vi "vacuum tray test.vi"() -> ()   [LabVIEW 2016]
uses:
  Classes/Controllers/I-O/Copy of NI-DAQ Folder/NI-DAQ.lvclass
  D:/INTT/V1/Classes/Controllers/I-O/Copy of I-O Folder/I-O.lvclass
  Classes/Controllers/I-O/Copy of I-O Folder/I-O.lvclass
panel:
  in  "stop":bool
  in  "Values":bool[](array[boolean])=[FALSE, FALSE]
  in  "TrayVaccum":bool
  in  "sampel vacuum":i32[](array[numeric])=[15, 19]
  out "vacuum on?":bool[](array[boolean])
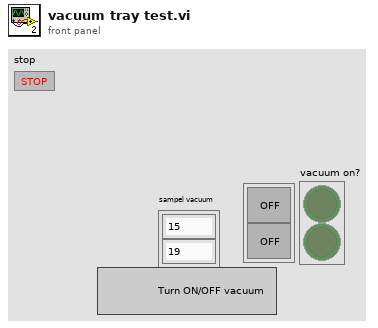
[diagram p1: front panel]
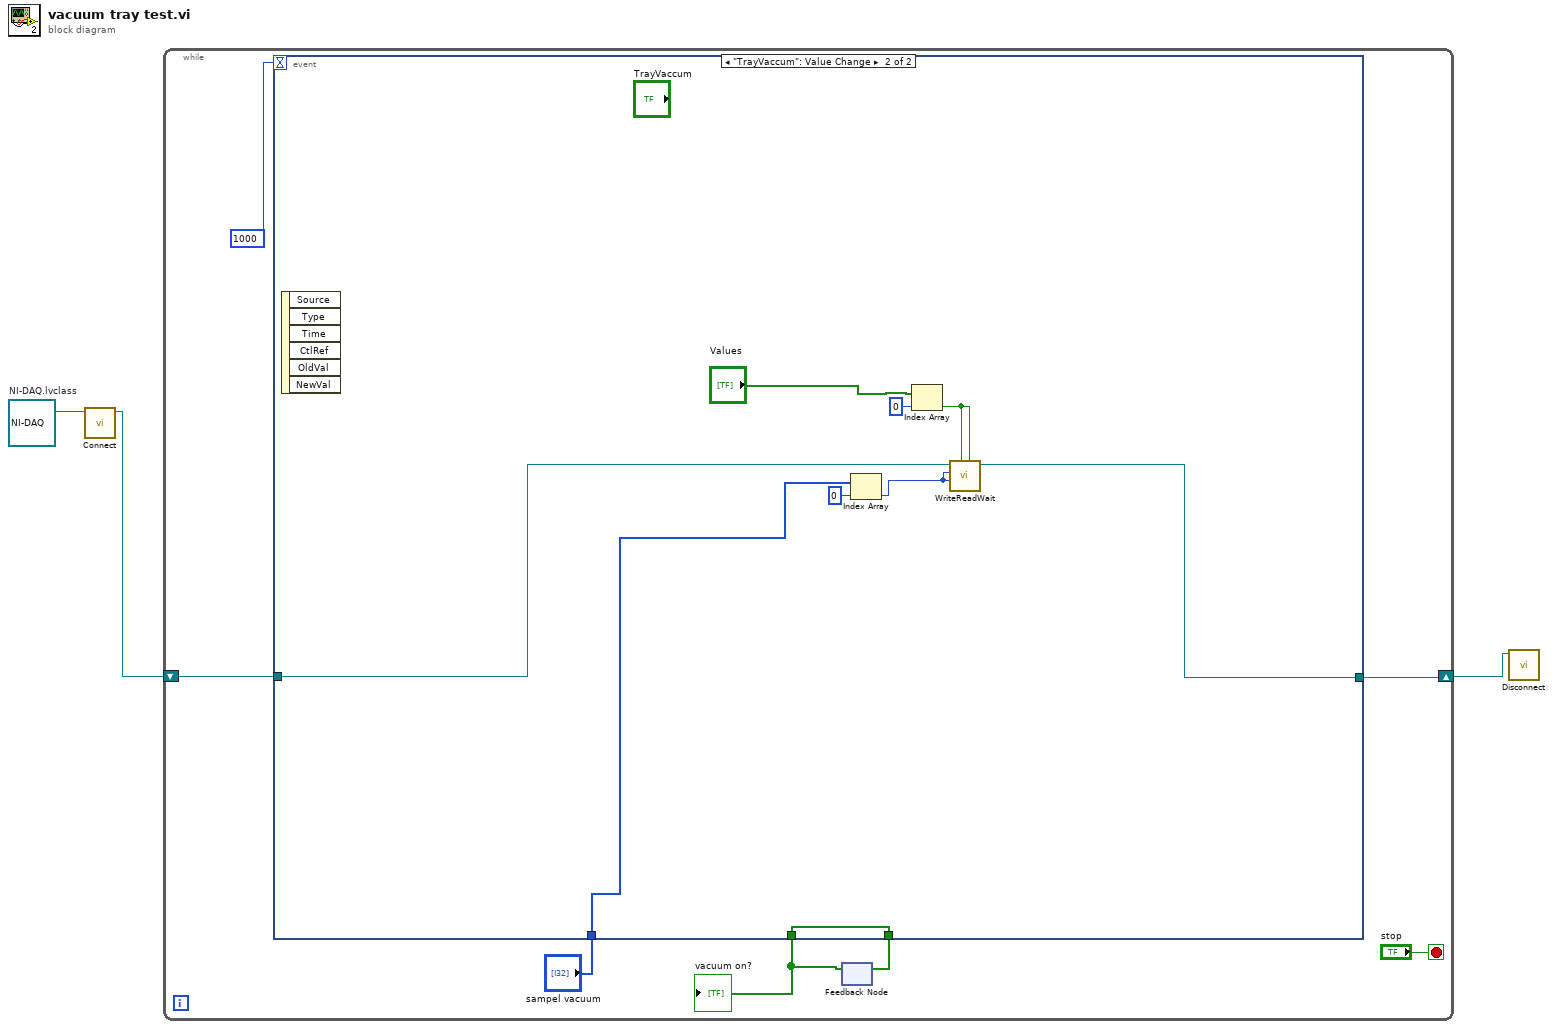
[diagram p0: block diagram]
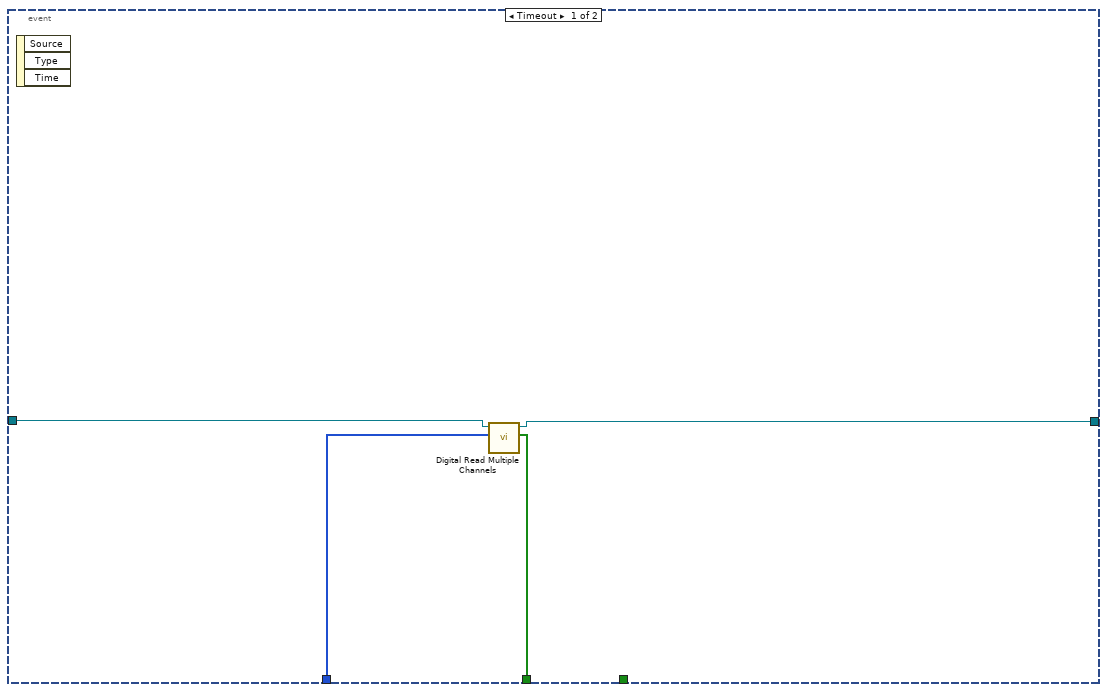
[diagram p2: hidden frame]
diagram:
  w3 = refnum<class "NI-DAQ.lvclass"> refnum  # NI-DAQ.lvclass
  n1 = call-dynamic "Connect.vi"("NI-DAQ in"=w3) -> ("NI-DAQ out"=w2:refnum<class "NI-DAQ.lvclass">)  [unwired: 9 in, 1 out]
  n2 = while {
    shift-right: [w7] -> w1
    shift-left: w2 -> [w8]
    stop <- "stop" stop-if-true
    n3 = feedback #1() -> (w4:bool[])  [unwired: 1 in]
    n4 = event shown="[1] \"TrayVaccum\": Value Change" {
      selector: _ -> [_ _]
      dyn-events: _ -> [_ _]
      timeout: 1000 -> [_ _]
      tunnel: w8 -> [w14 w16]
      tunnel: [w13 w15] -> w7
      tunnel: "sampel vacuum" -> [w12 w17]
      tunnel: [w11 w18] -> w5
      tunnel: w4 -> [_ w18]
      event Timeout {
        n5 = event-data() -> ()  [unwired: 1 in, 3 out]
        n6 = call-dynamic "Digital Read Multiple Channels.vi"("Array"=w12, "NI-DAQ in"=w14) -> ("subarray"=w11:bool[], "NI-DAQ out"=w13:refnum<class "NI-DAQ.lvclass">)  [unwired: 7 in, 1 out]
      }
      event "TrayVaccum": Value Change {
        n7 = event-data() -> ()  [unwired: 1 in, 6 out]
        n8 = Index Array(array=w17, index=0) -> (element=w22:i32)
        n9 = Index Array(array="Values", index=0) -> (element=w20:bool)
        n10 = call "WriteReadWait.vi"("Read Value"=w20, "Write Value"=w20, "Read"=w22, "Write"=w22, "I-O in"=w16) -> ("I-O out"=w15:refnum<class "NI-DAQ.lvclass">)  [unwired: 5 in, 1 out]
      }
    }
    "vacuum on?" <- w5
    n11 = feedback-in #1(w5) -> ()
  }
  n12 = call-dynamic "Disconnect.vi"("I-O in"=w1) -> ()  [unwired: 9 in, 1 out]
